vi "GetAbsTargetPos.vi"(4 "error in (no error)":errorcluster, 5 "Motor":i32, 6 "DeviceKey In":string, 7 "CmdLib In":refnum<k24>) -> (0 "error out":errorcluster, 1 "Target Pos":i32, 2 "DeviceKey Out":string, 3 "CmdLib Out":refnum<k24>)   [LabVIEW 2009]
uses:
  C:/Code/Apps/Utilities/Picomotor/PicomotorApp/Install/Samples/LabVIEW/Model 8742/LabVIEW 2009/CmdLib.dll
panel:
  in  "pos":i32
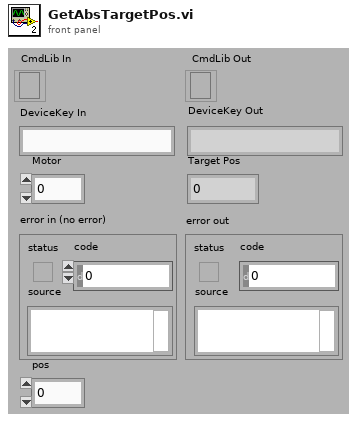
[diagram p1: front panel]
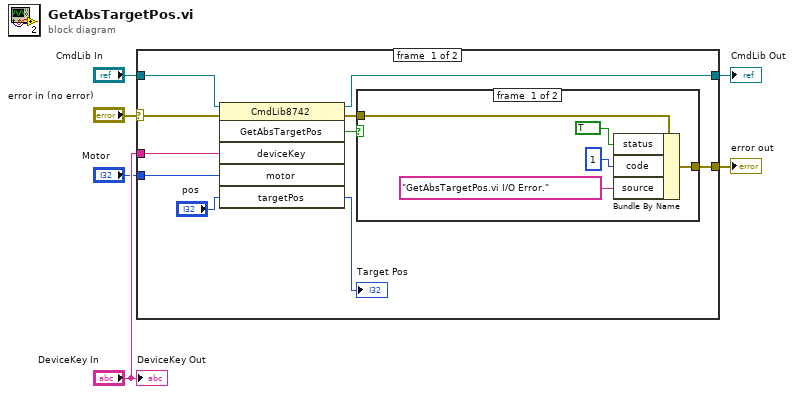
[diagram p0: block diagram]
diagram:
  n1 = case shown="No Error" "error in (no error)" {
    selector: "error in (no error)" -> [w12 w23]
    tunnel: "CmdLib In" -> [w16 w24]
    tunnel: [w15 w24] -> w5
    tunnel: "Motor" -> [w14 _]
    tunnel: "DeviceKey In" -> [w13 _]
    tunnel: [w9 w23] -> w2
    frame #0 {
      n2 = invoke class="CmdLib8742" method="GetAbsTargetPos"(reference=w16, error in=w12, "deviceKey"=w13, "motor"=w14, "targetPos"="pos") -> (reference out=w15:refnum<k24>, error out=w10:errorcluster, "GetAbsTargetPos"=w11:bool, "targetPos"=→"Target Pos":i32)  [unwired: 1 in, 2 out]
      n3 = case shown="False" w11 {
        tunnel: w10 -> [w21 w22]
        tunnel: [w20 w22] -> w9
        frame #0 {
          n4 = Bundle By Name(cluster=w21, "status"=TRUE, "code"=1, "source"="GetAbsTargetPos.vi I/O Error.") -> (w20:errorcluster)
        }
        frame #1 {
        }
      }
    }
    frame #1 {
    }
  }
  "error out" <- w2
  "CmdLib Out" <- w5
  "DeviceKey Out" <- "DeviceKey In"
